vi "Begin.vi"(8 "error in (no error)":errorcluster, 11 "Hatch Concrete in":refnum<class "Hatch Concrete.lvclass">) -> (0 "error out":errorcluster, 3 "Hatch Concrete out":refnum<class "Hatch Concrete.lvclass">)   [LabVIEW 2018, in "Hatch.lvlib" / "Hatch Concrete.lvclass"]
uses:
  Hatch Concrete.lvclass
  Hatch.lvclass
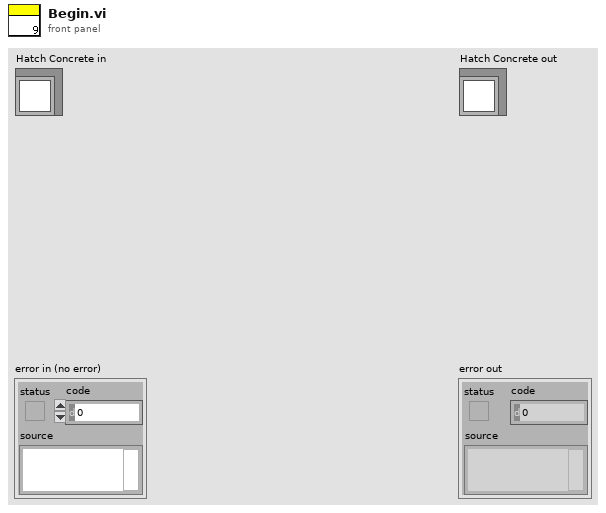
[diagram p1: front panel]
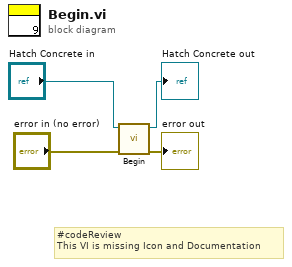
[diagram p0: block diagram]
diagram:
  # "#codeReview\nThis VI is missing Icon and Documentation"
  n1 = call-parent "Begin.vi"("error in (no error)"="error in (no error)", "Hatch in"="Hatch Concrete in") -> ("error out"=→"error out":errorcluster, "Hatch out"=→"Hatch Concrete out":refnum<class "Hatch Concrete.lvclass">)  [unwired: 8 in]
